vi "Find some Public API VI.vi"(8 "Framework VI to Find":T1, 9 "Library in":refnum<vi>, 10 "Target":refnum<vi>, 11 "App Ref":refnum<vi>) -> ()   [LabVIEW 2019, in "Panther Dashboard.lvlib"]
uses:
  Panther Dashboard.lvlib
  Public VIs names--enum.ctl
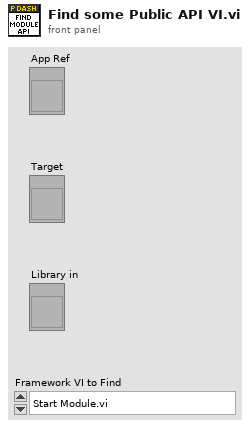
[diagram p1: front panel]
types:
  T1 = typedef "Panther Dashboard.lvlib/Public VIs names--enum.ctl" = enum16{"Start Module.vi", "Synchronize Module Events.vi", "Obtain Broadcast Events for Registration.vi", "Null Broadcast Events--constant.vi", "Stop Module.vi"}
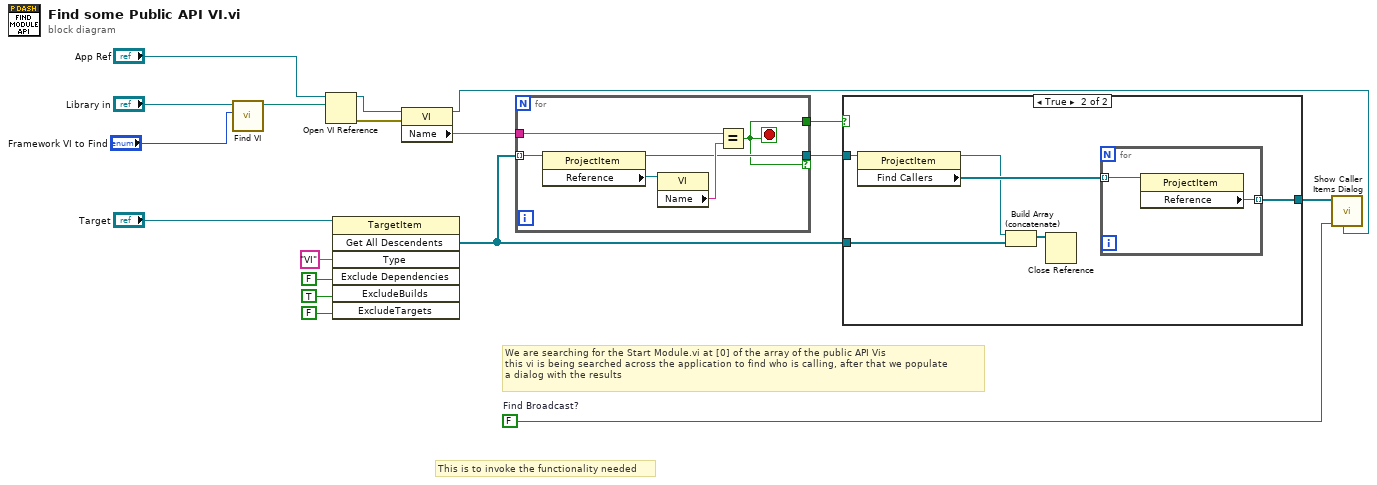
[diagram p0: block diagram]
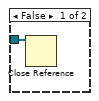
[diagram p2: hidden frame]
diagram:
  w2 = FALSE  # Find Broadcast?
  # "This is to invoke the functionality needed"
  # "We are searching for the Start Module.vi at [0] of the array of the public API Vis\nthis vi is being searched across the application to find who is calling, after that we populate\na dialog with the results"
  n1 = call "Find VI.vi"("Framework VI to Find"="Framework VI to Find", "Library in"="Library in") -> ("Framework VI Path"=w5:path)  [unwired: 9 in]
  n2 = Open VI Reference(application reference (local)="App Ref", vi path=w5) -> (vi reference=w7:refnum<vi>, error out=w18:errorcluster)  [unwired: 4 in]
  n3 = invoke class="TargetItem" method="Get All Descendents"(reference="Target", "Type"="VI", "Exclude Dependencies"=FALSE ("ExcludeDependencies"), "ExcludeBuilds"=TRUE, "ExcludeTargets"=FALSE) -> ("All Descendents"=w8:refnum<vi>[])  [unwired: 2 in, 6 out]
  n4 = property class="VI"(reference=w7, error in=w18) -> (reference out=w1:refnum<vi>, "Name"=w15:string)  [unwired: 1 out]
  n5 = for {
    tunnel: w8 -> [w24] mode=indexing
    tunnel: w15 -> [w21]
    tunnel: [w20] -> w13 if=w19
    tunnel: [w19] -> w14
    stop <- w19 stop-if-true
    n6 = property class="ProjectItem"(reference=w24) -> (reference out=w20:refnum<vi>, "Reference"=w23:refnum<vi>)  [unwired: 1 in, 1 out]
    n7 = property class="VI"(reference=w23) -> ("Name"=w22:string)  [unwired: 1 in, 2 out]
    n8 = Equal?(x=w21, y=w22) -> (x = y?=w19:bool)
  }
  n9 = case shown="True" w14 {
    tunnel: w13 -> [_ w31]
    tunnel: w8 -> [w25 w27]
    tunnel: [_ w29] -> w3
    frame False {
      n10 = Close Reference(reference=w25) -> ()  [unwired: 1 in, 1 out]
    }
    frame True {
      n11 = property class="ProjectItem"(reference=w31) -> (reference out=w28:refnum<vi>, "Find Callers"=w30:refnum<vi>[])  [unwired: 1 in, 1 out]
      n12 = Build Array (concatenate)(w28, w27) -> (w26:refnum<vi>[])
      n13 = Close Reference(reference=w26) -> ()  [unwired: 1 in, 1 out]
      n14 = for {
        tunnel: w30 -> [w33] mode=indexing
        tunnel: [w32] -> w29 mode=indexing
        n15 = property class="ProjectItem"(reference=w33) -> ("Reference"=w32:refnum<vi>)  [unwired: 1 in, 2 out]
      }
    }
  }
  n16 = call "Show Caller Items Dialog.vi"("Event"=w1, "Find Broadcast?"=w2, "Request VI Callers"=w3) -> ()  [unwired: 9 in]
